vi "GMLAN WriteDataByIdentifier.vi"(8 "error in (no error)":errorcluster, 9 "data":u8[](array[numeric]) format="%.0x", 10 "Data ID (DID)":u8 format="%.0x", 11 "diag ref in":T1) -> (0 "error out":errorcluster, 1 "success?":bool, 3 "diag ref out":T1)   [LabVIEW 2015, in "GMLAN.lvlib"]
uses:
  GMLAN.lvlib
  <vilib>/Automotive Diagnostic Command Set/Diagnostic Transport.llb/Diag Reference.ctl
  <vilib>/Automotive Diagnostic Command Set/Diagnostic Transport.llb/Transport Protocol Selector.ctl
  <vilib>/Automotive Diagnostic Command Set/Diagnostic Transport.llb/Diag CAN Frame Log.ctl
  <vilib>/addons/Automotive Diagnostic Command Set/NI_Automotive Diagnostic Command Set.lvlib
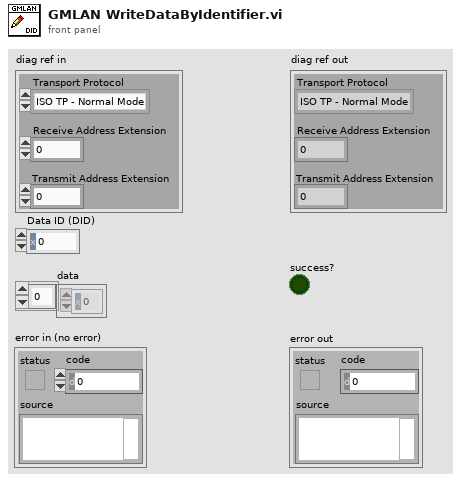
[diagram p1: front panel]
types:
  T1 = typedef "NI_Automotive Diagnostic Command Set.lvlib/Diag Reference.ctl" = cluster{"Diag CAN Handle":u32, "Transport Protocol":T2, "Receive Address Extension":u8, "Transmit Address Extension":u8, "Receive CAN Id":u32, "Transmit CAN Id":u32, "Diag CAN Queue":refnum<queue>, "Log Frames ?":bool, "My TP Address":u8, "Other TP Address":u8, "T1":u16, "T2":u16, "T3":u16, "T4":u16, "Tx SN":u8, "Block Size":u8, "Rx SN":u8, "VW TP Initialized?":bool, "Tx block no":u8, "baud rate":u32, "Interface":string, "Channel Diag CAN Handle":u32, "UDP Connection ID":refnum<k16>, "TCP Connection ID":refnum<k5>, "Target IP Addr":u32, "Source Address":u16, "Target Address":u16, "Send Header NACK?":bool, "DLL Handle":u32, "NAD":u8, "Time Stamp read first":dbl, "Time Stamp read last":dbl, "Time Stamp write first":dbl, "Time Stamp write last":dbl, "Time Stamp write":dbl, "Time Stamp read":dbl}
  T2 = typedef "NI_Automotive Diagnostic Command Set.lvlib/Transport Protocol Selector.ctl" = enum16{"ISO TP - Normal Mode", "ISO TP - Mixed Mode", "VW TP 2.0", "Diagnostics on IP", "ISO TP LIN"}
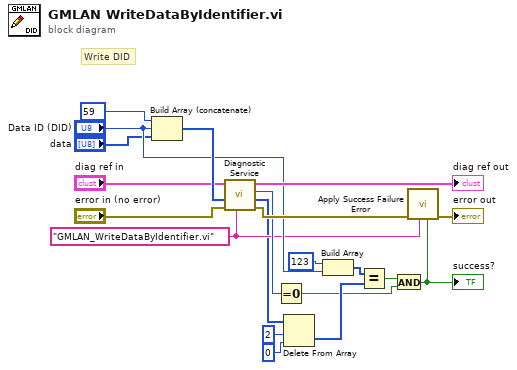
[diagram p0: block diagram]
diagram:
  w3 = "GMLAN_WriteDataByIdentifier.vi" ("error source")
  # "Write DID"
  n1 = Build Array (concatenate)(u8 59 ("element"), "Data ID (DID)", "data") -> (w16:u8[])
  n2 = call <vilib>:"Diagnostic Service.vi"("error source"=w3, "error in (no error)"="error in (no error)", "data in"=w16, "diag ref in"="diag ref in") -> ("error out"=w18:errorcluster, "data out"=w2:u8[], "error code"=w14:u8, "diag ref out"=→"diag ref out":T1)  [unwired: 2 in, 2 out]
  n3 = Equal To 0?(x=w14) -> (x = 0?=w8:bool)
  n4 = Delete From Array(array=w2, length=2, index=0) -> (deleted portion=w9:u8[])  [unwired: 1 out]
  n5 = Build Array(u8 123 ("element"), "Data ID (DID)") -> (w10:u8[])
  n6 = Equal?(x=w10, y=w9) -> (x = y?=w7:bool)
  n7 = And(x=w7, y=w8) -> (x .and. y?=w4:bool)
  "success?" <- w4
  n8 = call <vilib>:"Apply Success Failure Error.vi"("success code"=w4, "error source"=w3, "error in (no error)"=w18) -> ("error out"=→"error out":errorcluster)  [unwired: 8 out]
